vi "IOcard_analog_input_Meilhaus.vi"(10 "Channel":i32, 11 "Device":i32) -> (3 "Voltage [V]":dbl format="%.3f")   [LabVIEW 2009]
panel:
  in  "Trigger Edge":T1(ring)=enum."Any"
  in  "Trigger Type":T2(ring)=enum."Software"
  in  "Time Out [ms]":i32=5000
  out "Minimum Physical Range":dbl=-10.0 format="%.3f"
  out "Maximum Physical Range":dbl=9.999695 format="%.3f"
  out "Maximum Data Range":i32=65535
  in  "Minimum Physical Value":dbl=-10.0 format="%.2f"
  in  "Maximum Physical Value":dbl=9.99 format="%.2f"
  in  "Number of Channels":i32=32
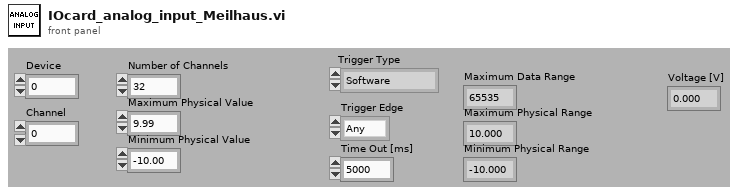
[diagram p1: front panel]
types:
  T1 = enum16{"None", "Above", "Below", "Entry", "Exit", "Rising", "Falling", "Any"}
  T2 = enum16{"None", "Software", "Threshold", "Window", "Edge", "Slope", "External Digital", "External Analog", "Pattern", "Timer", "Count", "Follow"}
  T3 = enum32{"Invalid", "Single", "Streaming", "Counter 8254", "Any"}
  T4 = enum32{"Invalid", "Analog Output", "Analog Input", "Digital I/O", "Digital Output", "Digital Input", "Counter", "External Interrupt"}
  T5 = cluster{"Device":i32, "Subdevice":i32, "Channel":i32, "Direction":i32, "Value":i32, "Time Out":i32, "Flags":i32, "Error":i32}[]
  T6 = cluster{"Device":i32, "Subdevice":i32, "Channel":i32, "Direction":i32, "Value":i32, "Time Out":i32, "Flags":i32, "Error Number":i32}[]
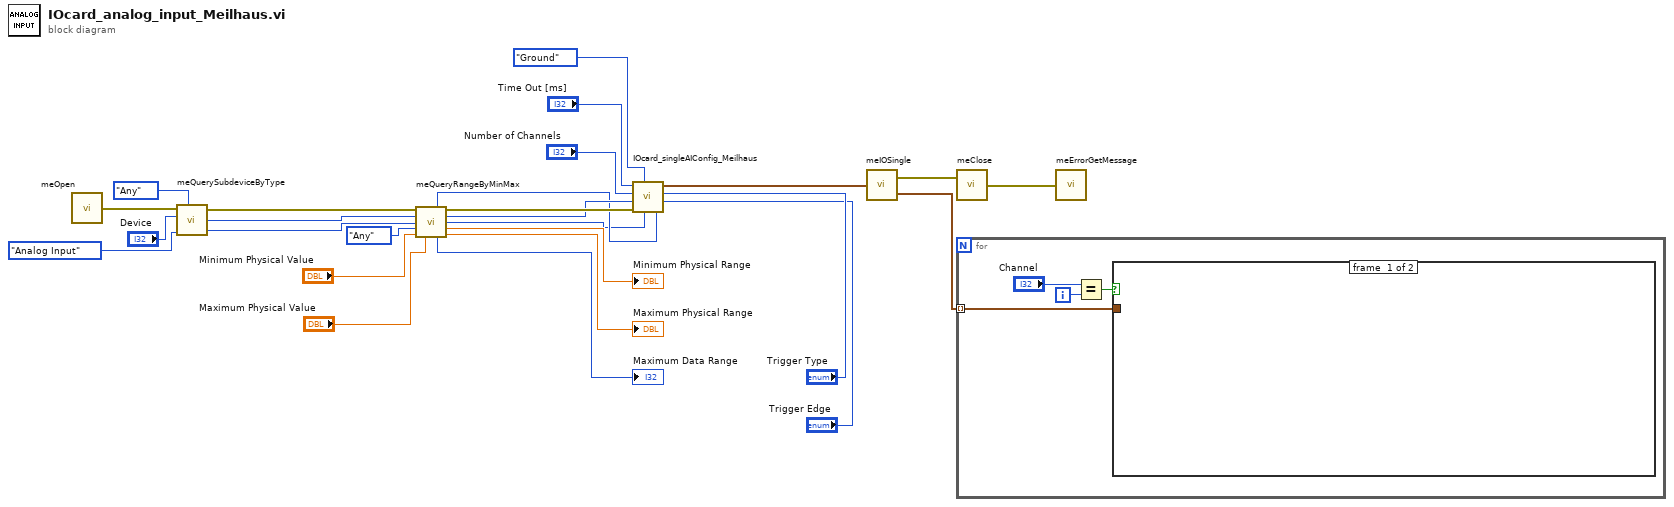
[diagram p0: block diagram]
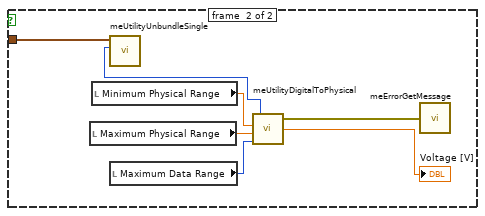
[diagram p2: hidden frame]
diagram:
  n1 = call <userlib>:"meOpen.vi"() -> ("error out"=w21:errorcluster)  [unwired: 2 in]
  n2 = call <userlib>:"meQuerySubdeviceByType.vi"("error in (no error)"=w21, "Device"="Device", "Type"=T4."Analog Input", "Subtype"=T3."Any") -> ("error out"=w18:errorcluster, "Device"=w17:i32, "Subdevice"=w16:i32)  [unwired: 1 in]
  n3 = call <userlib>:"meQueryRangeByMinMax.vi"("error in (no error)"=w18, "Device"=w17, "Subdevice"=w16, "Unit"=enum16{"Invalid", "Volt", "Ampere", "Any"}."Any", "Minimum Physical Value"="Minimum Physical Value", "Maximum Physical Value"="Maximum Physical Value") -> ("Range"=w10:i32, "error out"=w12:errorcluster, "Device"=w11:i32, "Subdevice"=w2:i32, "Minimum Physical Range"=→"Minimum Physical Range":dbl, "Maximum Data Range"=→"Maximum Data Range":i32, "Maximum Physical Range"=→"Maximum Physical Range":dbl)  [unwired: 3 in]
  n4 = call "IOcard_singleAIConfig_Meilhaus.vi"("Range"=w10, "Trigger Edge"="Trigger Edge", "Trigger Type"="Trigger Type", "Subdevice"=w2, "AI Reference"=enum16{"Ground", "Differential"}."Ground", "Error input"=w12, "Device"=w11, "Number of Channels"="Number of Channels", "Time Out"="Time Out [ms]") -> ("Array"=w26:T5)
  n5 = call <userlib>:"meIOSingle.vi"("Single List"=w26) -> ("Single List"=w22:T6, "error out"=w24:errorcluster)  [unwired: 2 in]
  n6 = call <userlib>:"meClose.vi"("error in (no error)"=w24) -> ("error out"=w1:errorcluster)  [unwired: 1 in]
  n7 = for {
    tunnel: w22 -> [w30] mode=indexing
    i -> [w28]
    n8 = Equal?(x="Channel", y=w28) -> (x = y?=w29:bool)
    n9 = case shown="True" w29 {
      tunnel: w30 -> [_ w36]
      frame #0 {
      }
      frame #1 {
        n10 = local read "Maximum Physical Range"() -> (w33:dbl)
        n11 = local read "Minimum Physical Range"() -> (w34:dbl)
        n12 = call <userlib>:"meUtilityUnbundleSingle.vi"("Single Entry"=w36) -> ("Value"=w35:i32)  [unwired: 6 out]
        n13 = local read "Maximum Data Range"() -> (w32:i32)
        n14 = call <userlib>:"meUtilityDigitalToPhysical.vi"("Data"=w35, "Minimum Pyhsical Value"=w34, "Maximum Pysical Value"=w33, "Maximum Digital Data"=w32) -> ("error out"=w37:errorcluster, "Physical Value"=→"Voltage [V]":dbl)  [unwired: 3 in]
        n15 = call <userlib>:"meErrorGetMessage.vi"("error in (no error)"=w37) -> ()
      }
    }
  }
  n16 = call <userlib>:"meErrorGetMessage.vi"("error in (no error)"=w1) -> ()
